vi "SLL DE Unit Info LV2Global.vi"(6 "Option":T5=enum."Read", 7 "Units Information":T3(array[cluster]), 8 "Error in (no error)":errorcluster, 9 "AI Channel Type":T1[](array[typedef]), 10 "AI Channel Names":T4[](array[typedef]), 11 "Channel Name":string) -> (0 "Error out":errorcluster, 2 "Unit Info":T2, 3 "Valid?":bool)   [LabVIEW 2009]
uses:
  Controls/SLL DE Unit Info LV2Global Options.ctl
  Controls/SLL DE List of Analog Inputs.ctl
  Controls/SLL DE List of AI Channel Type.ctl
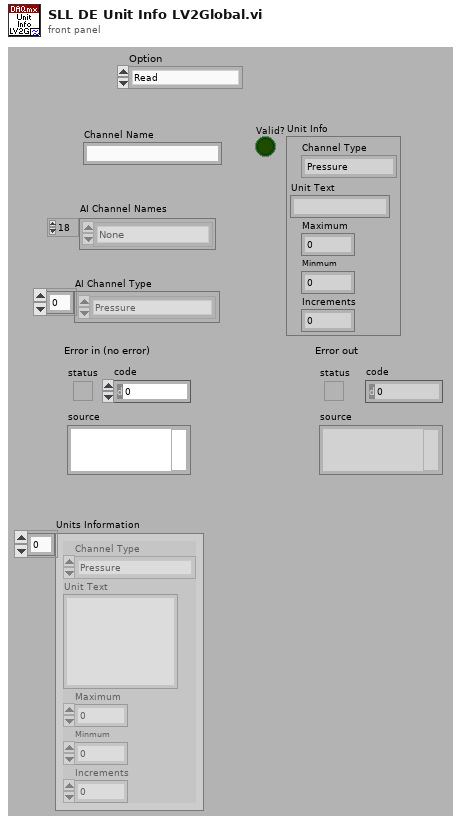
[diagram p1: front panel]
types:
  T1 = typedef "SLL DE List of AI Channel Type.ctl" = enum16{"Pressure", "Flow", "Temperature", "Time Scale", "Voltage", "Current", "Frequency", "Sound", "Speed", "Torque", "Distance", "Channel Type 1", "Channel Type 2", "Channel Type 3"}
  T2 = cluster{"Channel Type":T1, "Unit Text":string, "Maximum":dbl, "Minmum":dbl, "Increments":dbl}
  T3 = cluster{"Channel Type":T1, "Unit Text":string, "Maximum":dbl, "Minmum":dbl, "Increments":dbl}[]
  T4 = typedef "SLL DE List of Analog Inputs.ctl" = enum16{"None"}
  T5 = typedef "SLL DE Unit Info LV2Global Options.ctl" = enum16{"Update Channel Type", "Update Unit Info", "Get Unit Info", "Read"}
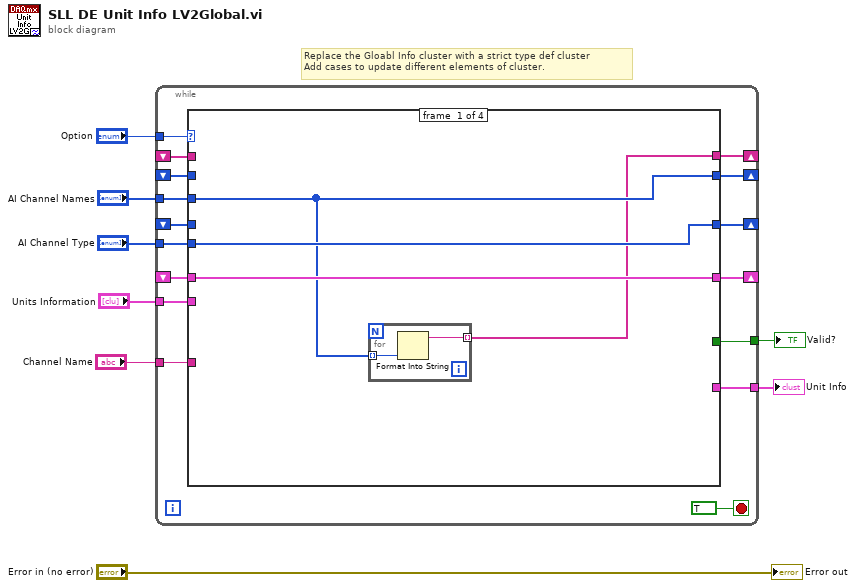
[diagram p0: block diagram]
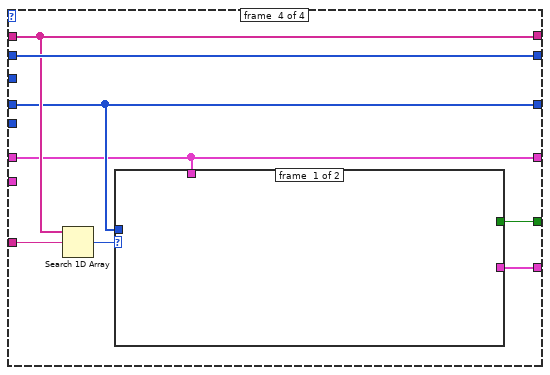
[diagram p4: hidden frame]
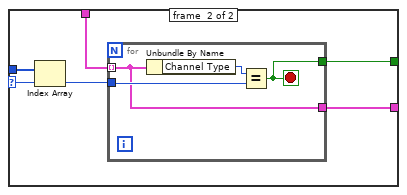
[diagram p5: hidden frame]
diagram:
  # "Replace the Gloabl Info cluster with a strict type def cluster\nAdd cases to update different elements of cluster."
  n1 = while {
    tunnel: "Option" -> [w23]
    tunnel: "AI Channel Names" -> [w22]
    tunnel: "AI Channel Type" -> [w21]
    tunnel: "Units Information" -> [w20]
    shift-right: [w19] -> _
    shift-left: _ -> [w18]
    shift-right: [w17] -> _
    shift-left: _ -> [w16]
    shift-right: [w15] -> _
    shift-left: _ -> [w14]
    tunnel: "Channel Name" -> [w13]
    shift-right: [w12] -> _
    shift-left: _ -> [w11]
    tunnel: [w10] -> w2
    tunnel: [w9] -> w1
    stop <- TRUE stop-if-true
    n2 = case shown="\"Get Unit Info\"" w23 {
      tunnel: w22 -> [w26 _ _ _]
      tunnel: w21 -> [w28 _ _ _]
      tunnel: w20 -> [_ w32 _ _]
      tunnel: [w26 w33 w38 w46] -> w19
      tunnel: w18 -> [_ w33 w38 w46]
      tunnel: [w28 w34 w37 w42] -> w17
      tunnel: w16 -> [_ w34 w37 w42]
      tunnel: [w27 w32 w36 w41] -> w15
      tunnel: w14 -> [w27 _ w36 w41]
      tunnel: w13 -> [_ _ _ w44]
      tunnel: [w25 w31 w35 w45] -> w12
      tunnel: w11 -> [_ w31 w35 w45]
      tunnel: [_ _ _ w40] -> w10
      tunnel: [_ _ _ w39] -> w9
      frame #0 {
        n3 = for {
          tunnel: w26 -> [w30] mode=indexing
          tunnel: [w29] -> w25 mode=indexing
          n4 = Format Into String(w30) -> (resulting string=w29:string)  [unwired: 3 in, 1 out]
        }
      }
      frame #1 {
      }
      frame #2 {
      }
      frame #3 {
        n5 = Search 1D Array(1D array=w45, element=w44) -> (index of element=w43:i32)  [unwired: 1 in]
        n6 = case shown="Default" w43 {
          selector: w43 -> [_ w52]
          tunnel: w42 -> [_ w51]
          tunnel: w41 -> [_ w49]
          tunnel: [_ w48] -> w40
          tunnel: [_ w47] -> w39
          frame #0 {
          }
          frame #1 {
            n7 = Index Array(array=w51, index=w52) -> (element=w50:T1)
            n8 = for {
              tunnel: w50 -> [w56]
              tunnel: w49 -> [w54] mode=indexing
              tunnel: [w54] -> w47
              tunnel: [w53] -> w48
              stop <- w53 stop-if-true
              n9 = Unbundle By Name(w54) -> ("Channel Type"=w55:T1)
              n10 = Equal?(x=w55, y=w56) -> (x = y?=w53:bool)
            }
          }
        }
      }
    }
  }
  "Valid?" <- w2
  "Unit Info" <- w1
  "Error out" <- "Error in (no error)"
